vi "Pre-Uninstall Custom Action.vi"(10 "Variant":variant) -> (0 "error out":errorcluster)   [LabVIEW 2014]
uses:
  <vilib>/zip/NI_Unzip.lvlib
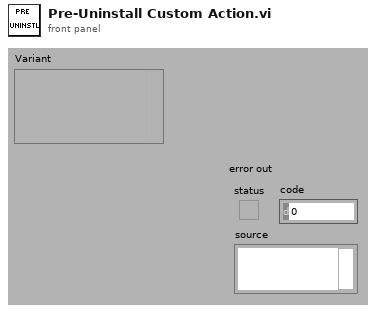
[diagram p1: front panel]
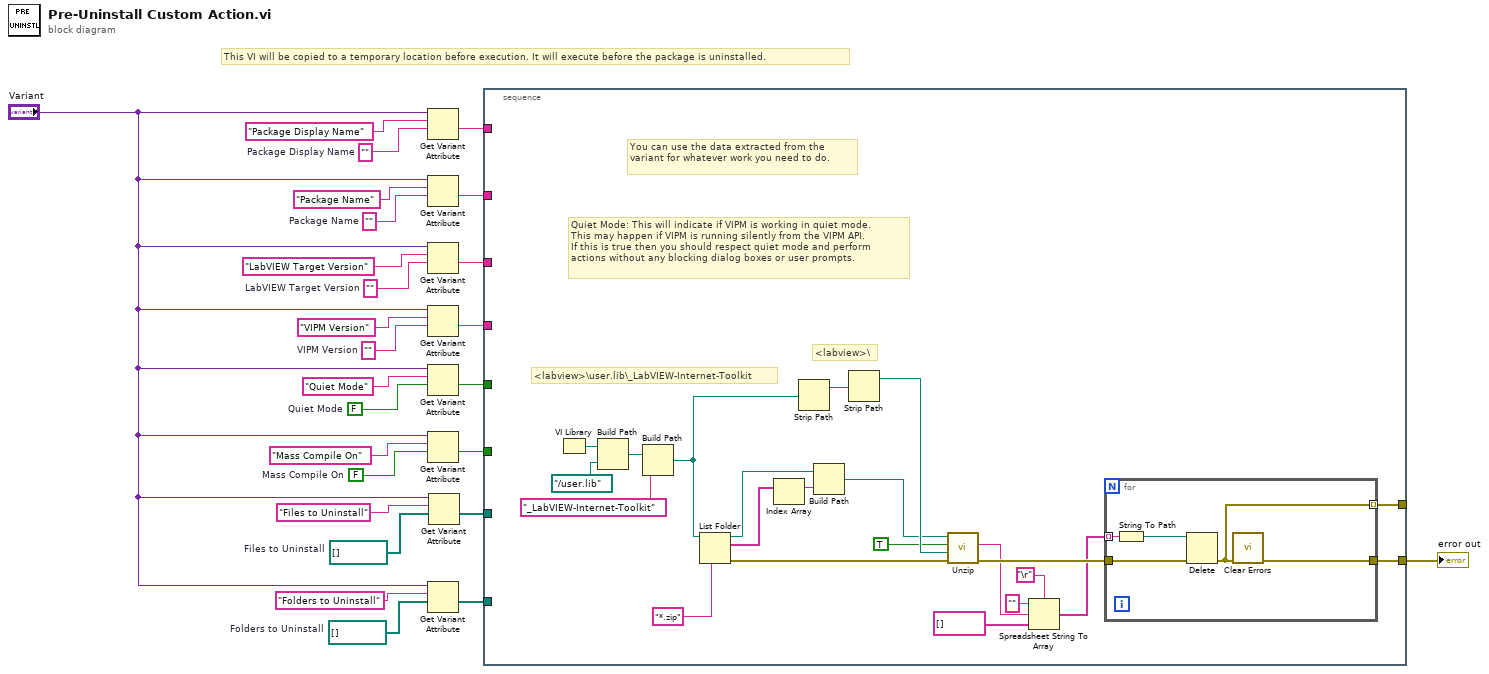
[diagram p0: block diagram]
diagram:
  w4 = path[] []  # Folders to Uninstall
  w8 = path[] []  # Files to Uninstall
  w9 = FALSE  # Mass Compile On
  w10 = ""  # Package Display Name
  w17 = FALSE  # Quiet Mode
  w20 = ""  # VIPM Version
  w22 = ""  # LabVIEW Target Version
  w24 = ""  # Package Name
  # "This VI will be copied to a temporary location before execution. It will execute before the package is uninstalled."
  n1 = Get Variant Attribute(Variant="Variant", name="Package Display Name", default value (empty Variant)=w10) -> (value=w16:string)  [unwired: 1 in, 3 out]
  n2 = Get Variant Attribute(Variant="Variant", name="Package Name", default value (empty Variant)=w24) -> (value=w15:string)  [unwired: 1 in, 3 out]
  n3 = Get Variant Attribute(Variant="Variant", name="LabVIEW Target Version", default value (empty Variant)=w22) -> (value=w14:string)  [unwired: 1 in, 3 out]
  n4 = Get Variant Attribute(Variant="Variant", name="VIPM Version", default value (empty Variant)=w20) -> (value=w13:string)  [unwired: 1 in, 3 out]
  n5 = Get Variant Attribute(Variant="Variant", name="Quiet Mode", default value (empty Variant)=w17) -> (value=w12:bool)  [unwired: 1 in, 3 out]
  n6 = Get Variant Attribute(Variant="Variant", name="Mass Compile On", default value (empty Variant)=w9) -> (value=w11:bool)  [unwired: 1 in, 3 out]
  n7 = Get Variant Attribute(Variant="Variant", name="Folders to Uninstall", default value (empty Variant)=w4) -> (value=w3:path[])  [unwired: 1 in, 3 out]
  n8 = Get Variant Attribute(Variant="Variant", name="Files to Uninstall", default value (empty Variant)=w8) -> (value=w6:path[])  [unwired: 1 in, 3 out]
  n9 = stacked-sequence {
    tunnel: w16 -> [_]
    tunnel: w15 -> [_]
    tunnel: w14 -> [_]
    tunnel: w13 -> [_]
    tunnel: w12 -> [_]
    tunnel: w11 -> [_]
    tunnel: w6 -> [_]
    tunnel: w3 -> [_]
    tunnel: [w38] -> w1
    tunnel: [w32] -> _
    frame #0 {
      # "<labview>\\"
      # "<labview>\\user.lib\\_LabVIEW-Internet-Toolkit"
      # "Quiet Mode: This will indicate if VIPM is working in quiet mode.\nThis may happen if VIPM is running silently from the VIPM API.\nIf this is true then you should respect quiet mode and perform\nactions without any blocking dialog boxes or user prompts."
      # "You can use the data extracted from the variant for whatever work you need to do."
      n10 = VI Library() -> (path=w30:path)
      n11 = Build Path(base path=w30, name or relative path=path "../user.lib" ("Relative path (.)")) -> (appended path=w29:path)
      n12 = Build Path(base path=w29, name or relative path="_LabVIEW-Internet-Toolkit") -> (appended path=w27:path)
      n13 = List Folder(path=w27, pattern="*.zip") -> (path out=w44:path, filenames=w43:string[], error out=w41:errorcluster)  [unwired: 2 in, 1 out]
      n14 = Index Array(array=w43) -> (element=w42:string)  [unwired: 1 in]
      n15 = Strip Path(path=w27) -> (stripped path=w48:path)  [unwired: 1 out]
      n16 = Build Path(base path=w44, name or relative path=w42) -> (appended path=w46:path)
      n17 = Strip Path(path=w48) -> (stripped path=w47:path)  [unwired: 1 out]
      n18 = call <vilib>:"Unzip.vi"("error in (no error)"=w41, "Target directory (same as Zip file if empty)"=w47, "Preview only?"=TRUE, "Zip file"=w46) -> ("error out"=w39:errorcluster, "Preview"=w37:string)  [unwired: 5 in, 1 out]
      n19 = Spreadsheet String To Array(delimiter (Tab)="\r", format string="", spreadsheet string=w37, array type (2D Dbl)=string[] []) -> (array=w35:string[])
      n20 = for {
        tunnel: w35 -> [w53] mode=indexing
        tunnel: w39 -> [w52]
        tunnel: [w51] -> w38
        tunnel: [w49] -> w32 mode=indexing
        n21 = String To Path(string=w53) -> (path=w50:path)
        n22 = Delete(path (use dialog)=w50, error in=w52) -> (error out=w49:errorcluster)  [unwired: 3 in, 2 out]
        n23 = call <vilib>:"Clear Errors.vi"("error in (no error)"=w49) -> ("error out"=w51:errorcluster)  [unwired: 5 in, 1 out]
      }
    }
  }
  "error out" <- w1
